vi "createNewExcelDocument.vi"(8 "error in (no error)":errorcluster, 10 "Excel File Path":path, 11 "xssfWorkbook in":refnum<class "xssfWorkbook.lvclass">) -> (0 "error out":errorcluster, 3 "xssfWorkbook out":refnum<class "xssfWorkbook.lvclass">)   [LabVIEW 2017, in "Excel_Specific.lvlib" / "xssfWorkbook.lvclass"]
uses:
  xssfWorkbook.lvclass
  C:/Users/Neo/Desktop/Dev_Tools_BR/LabVIEW_NPOI/src/LabVIEW NPOI/NPOI_Document/npoiDocument/npoiDocument.lvclass
  C:/Users/Neo/Desktop/Dev_Tools_BR/LabVIEW_NPOI/src/lib/NPOI 2.1.1/NPOI.OOXML.dll
  lib/NPOI 2.1.1/NPOI.OOXML.dll
  NPOI_Document/npoiDocument/npoiDocument.lvclass/npoiDocument.ctl
  NPOI_Document/npoiDocument/Get Document.Path.vi
  Support/File Stream/File Stream.lvlib
  NPOI_Document/npoiDocument/npoiDocument.lvclass
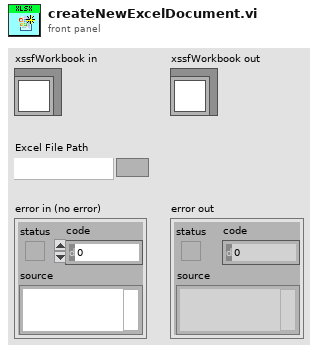
[diagram p1: front panel]
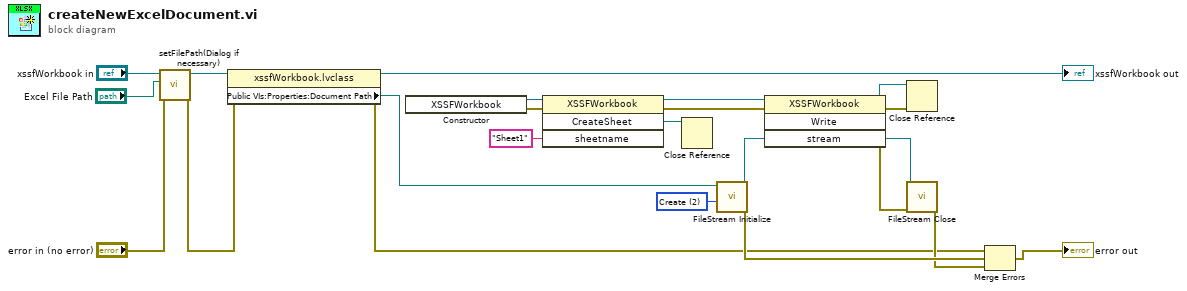
[diagram p0: block diagram]
diagram:
  w9 = 2 items=["CreateNew"=1, "Create"=2, "Open"=3, "OpenOrCreate"=4, "Truncate"=5, "Append"=6] ("mode")
  n1 = call "setFilePath(Dialog if necessary).vi"("error in (no error)"="error in (no error)", "File Path"="Excel File Path", "npoiDocument in"="xssfWorkbook in") -> ("error out"=w1:errorcluster, "npoiDocument out"=w4:refnum<class "xssfWorkbook.lvclass">)  [unwired: 7 in]
  n2 = property class="xssfWorkbook.lvclass"(reference=w4, error in=w1) -> (reference out=→"xssfWorkbook out":refnum<class "xssfWorkbook.lvclass">, error out=w8:errorcluster, "Public VIs:Properties:Document Path"=w15:path)
  n3 = constructor class="XSSFWorkbook"() -> (reference out=w20:refnum<k24>, error out=w21:errorcluster)  [unwired: 3 in, 1 out]
  n4 = invoke class="XSSFWorkbook" method="CreateSheet"(reference=w20, error in=w21, "sheetname"="Sheet1") -> (reference out=w18:refnum<k24>, error out=w16:errorcluster, "CreateSheet"=w14:refnum<k24>)  [unwired: 1 in, 1 out]
  n5 = Close Reference(reference=w14) -> ()  [unwired: 1 in, 1 out]
  n6 = call "FileStream Initialize.vi"("mode"=w9, "path"=w15) -> ("error out"=w13:errorcluster, "new reference"=w17:refnum<k24>)  [unwired: 8 in]
  n7 = invoke class="XSSFWorkbook" method="Write"(reference=w18, error in=w16, "stream"=w17) -> (reference out=w11:refnum<k24>, error out=w10:errorcluster)  [unwired: 1 in, 2 out]
  n8 = Close Reference(reference=w11, error in (no error)=w10) -> ()  [unwired: 1 out]
  n9 = call "FileStream Close.vi"("error in (no error)"=w10, "reference"=w17) -> ("error out"=w12:errorcluster)  [unwired: 9 in]
  n10 = Merge Errors(w8, w13, w12) -> (→"error out":errorcluster)
